vi "Enqueue Message.vi"(0 "Message Queue In":refnum<queue>, 5 "Message Id":string, 7 "Message Data":variant, 9 "Priority":bool, 11 "error in (no error)":errorcluster) -> (4 "Message Queue Out":refnum<queue>, 15 "error out":errorcluster)   [LabVIEW 2023, in "HAF.lvlib"]
doc: "Places a message on the given queue, at the front if a priority message."
uses:
  HAF.lvlib
  Message.ctl
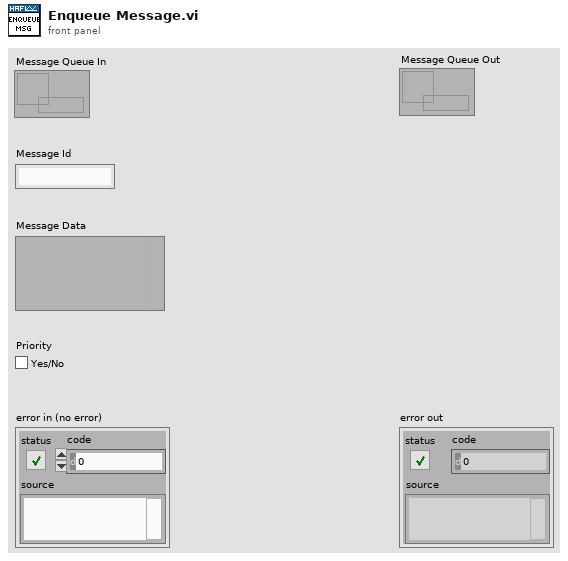
[diagram p1: front panel]
types:
  T1 = typedef "HAF.lvlib/Message.ctl" = cluster{"Message Id":string, "Message Data":variant}
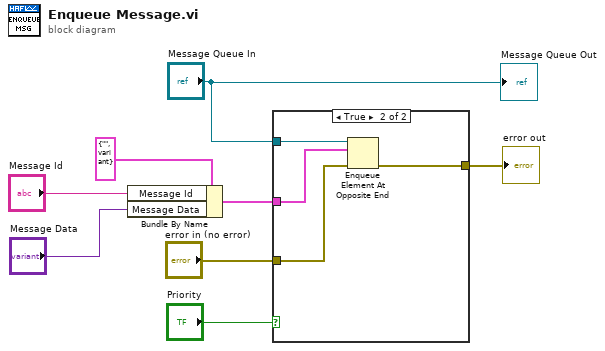
[diagram p0: block diagram]
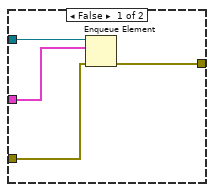
[diagram p2: hidden frame]
diagram:
  n1 = Bundle By Name(cluster=T1 {"Message Id"="", "Message Data"=variant} ("Message Structure"), "Message Id"="Message Id", "Message Data"="Message Data") -> (w3:T1)
  n2 = case shown="True" "Priority" {
    tunnel: "error in (no error)" -> [w10 w14]
    tunnel: "Message Queue In" -> [w12 w16]
    tunnel: w3 -> [w11 w15]
    tunnel: [w9 w13] -> w2
    frame False {
      n3 = Enqueue Element(queue=w12, element=w11, error in (no error)=w10) -> (error out=w9:errorcluster)  [unwired: 1 in, 2 out]
    }
    frame True {
      n4 = Enqueue Element At Opposite End(queue=w16, element=w15, error in (no error)=w14) -> (error out=w13:errorcluster)  [unwired: 1 in, 2 out]
    }
  }
  "error out" <- w2
  "Message Queue Out" <- "Message Queue In"
